vi "Inficon - Send command.vi"(8 "Error In":errorcluster, 10 "Command":string, 11 "COM in":refnum<visa-resource-name>) -> (0 "Error Out":errorcluster, 2 "Output":string, 3 "COM out":refnum<visa-resource-name>)   [LabVIEW 2016]
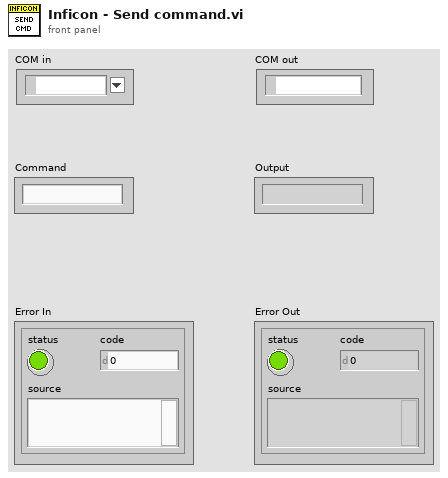
[diagram p1: front panel]
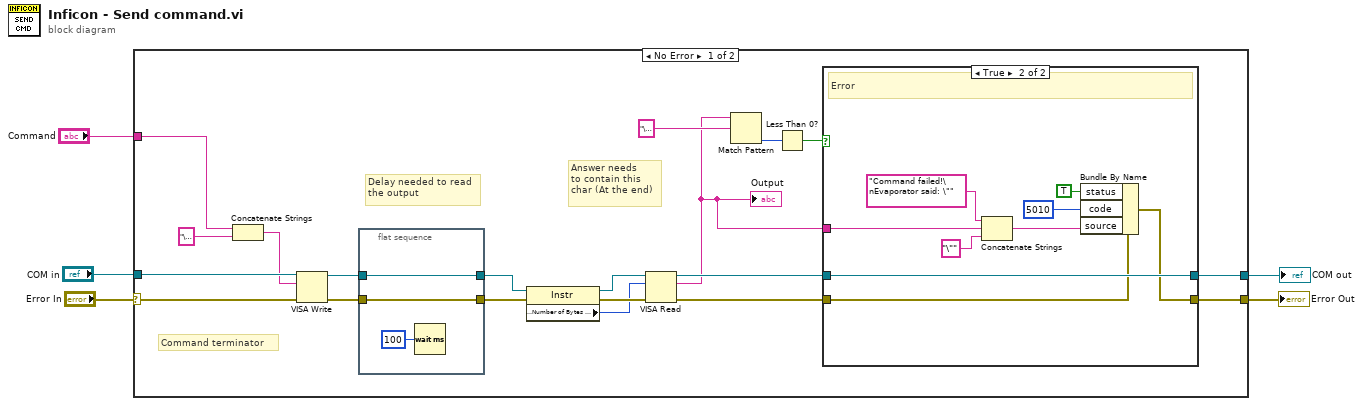
[diagram p0: block diagram]
diagram:
  n1 = case shown="No Error" "Error In" {
    selector: "Error In" -> [w24 w41]
    tunnel: [w11 w41] -> w4
    tunnel: "Command" -> [w15 _]
    tunnel: "COM in" -> [w16 w40]
    tunnel: [w13 w40] -> w1
    frame No Error {
      # "Answer needs \nto contain this\nchar (At the end)"
      # "Delay needed to read\nthe output"
      # "Command terminator"
      n2 = Concatenate Strings(w15, "\u0006") -> (w14:string)
      n3 = VISA Write(VISA resource name=w16, write buffer=w14, error in (no error)=w24) -> (VISA resource name out=w19:refnum<visa-resource-name>, error out=w20:errorcluster)  [unwired: 1 out]
      n4 = flat-sequence {
        tunnel: w20 -> [w37]
        tunnel: w19 -> [w38]
        tunnel: [w38] -> w18
        tunnel: [w37] -> w17
        frame #0 {
          n5 = Wait (ms)(milliseconds to wait=u32 100) -> ()  [unwired: 1 out]
        }
      }
      n6 = property class="Instr"(reference=w18, error in=w17) -> (reference out=w22:refnum<visa-resource-name>, error out=w23:errorcluster, "Serial Settings:Number of Bytes at Serial Port"=w21:u32)
      n7 = VISA Read(VISA resource name=w22, byte count=w21, error in (no error)=w23) -> (VISA resource name out=w12:refnum<visa-resource-name>, read buffer=w8:string, error out=w10:errorcluster)  [unwired: 1 out]
      "Output" <- w8
      n8 = Match Pattern(string=w8, regular expression="\u0006") -> (offset past match=w6:i32)  [unwired: 1 in, 3 out]
      n9 = Less Than 0?(x=w6) -> (x < 0?=w7:bool)
      n10 = case shown="True" w7 {
        tunnel: [w27 w36] -> w13
        tunnel: w12 -> [w27 w36]
        tunnel: [w26 w32] -> w11
        tunnel: w10 -> [w26 w31]
        tunnel: w8 -> [_ w34]
        frame False {
          # "No error"
        }
        frame True {
          # "Error"
          n11 = Concatenate Strings("Command failed!\nEvaporator said: \"" ("[error source] (\" \")"), w34, "\"" ("string")) -> (w28:string)
          n12 = Bundle By Name(cluster=w31, "status"=TRUE, "code"=5010 ("[error code] (0)"), "source"=w28) -> (w32:errorcluster)
        }
      }
    }
    frame Error {
    }
  }
  "COM out" <- w1
  "Error Out" <- w4
